vi "Error 5002.vi"(8 "error in (no error)":errorcluster) -> (2 "Emergency Stop":bool)   [LabVIEW 2019]
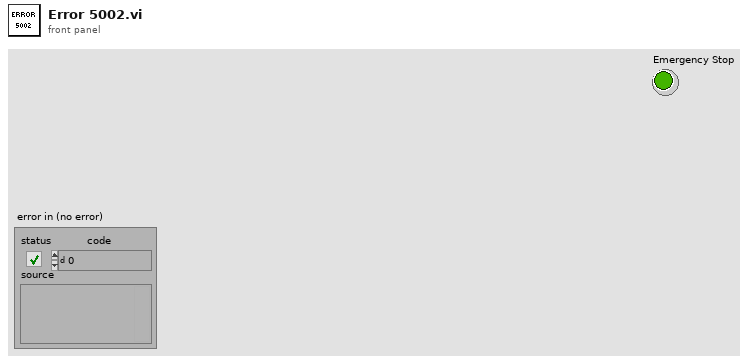
[diagram p1: front panel]
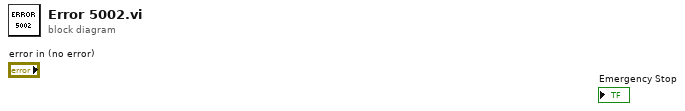
[diagram p0: block diagram]
diagram:
